vi "WFM_1D.vi"(4 "Value":waveform(dbl)[](array[waveform])) -> (1 "Constant":refnum<class "Const_WFM_1D.lvclass">)   [LabVIEW 2021, in "Const_WFM_1D.lvclass"]
uses:
  Const_WFM_1D.lvclass
  Const_WFM_1D.lvclass/Const_WFM_1D.ctl
  Properties/Write Value.vi
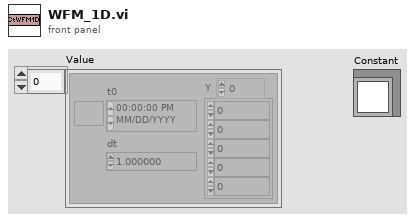
[diagram p1: front panel]
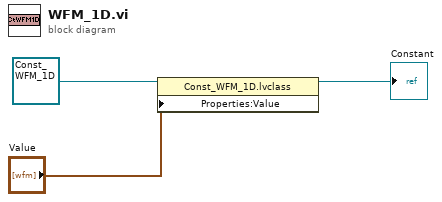
[diagram p0: block diagram]
diagram:
  n1 = property class="Const_WFM_1D.lvclass"(reference=refnum<class "Const_WFM_1D.lvclass"> refnum ("Constants.lvlib:Numeric.lvclass"), "Properties:Value"="Value") -> (reference out=→"Constant":refnum<class "Const_WFM_1D.lvclass">)  [unwired: 1 in, 1 out]
